vi "Map Image.vi"(2 "End of Canon highet [meters]":dbl, 3 "Goal Number":i32(knob) scale=1.0..5.0, 4 "Y[Pixels]":dbl, 5 "X [Pixels]":dbl) -> (0 "Distance [Meter]":dbl, 1 "Angel [Degrees]":dbl)   [LabVIEW 2012]
panel:
  out "Distance on ground [Meter]":dbl
  # "Goals Hights:\n1-high\n2-right\n3-left\n4-low\n5-pyramid"
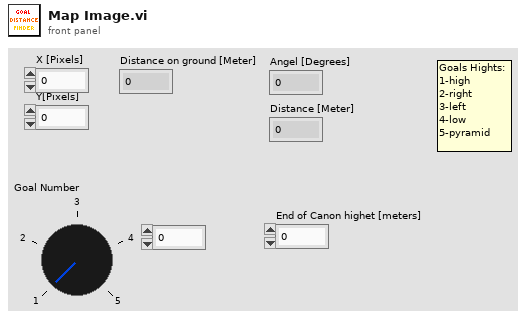
[diagram p1: front panel]
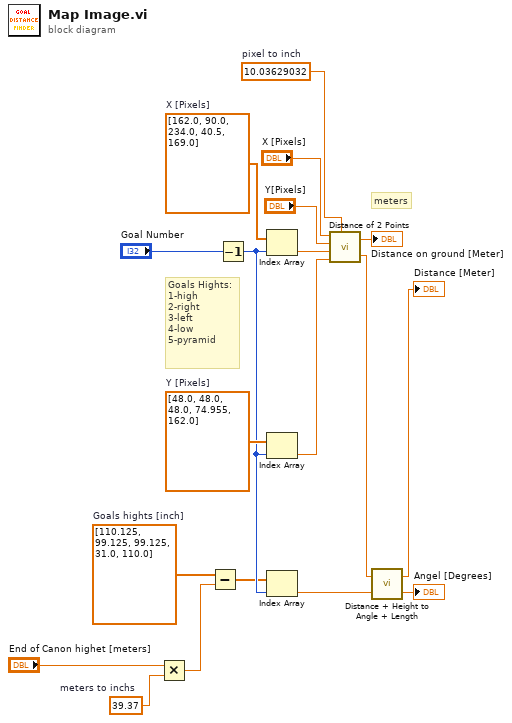
[diagram p0: block diagram]
diagram:
  w4 = 39.37  # meters to inchs
  w15 = dbl[] [48.0, 48.0, 48.0, 74.955, 162.0]  # Y [Pixels]
  w16 = dbl[] [162.0, 90.0, 234.0, 40.5, 169.0]  # X [Pixels]
  w3 = dbl[] [110.125, 99.125, 99.125, 31.0, 110.0]  # Goals hights [inch]
  w13 = 10.03629032  # pixel to inch
  # "Goals Hights:\n1-high\n2-right\n3-left\n4-low\n5-pyramid"
  # "meters"
  n1 = Multiply(x="End of Canon highet [meters]", y=w4) -> (x*y=w2:dbl)
  n2 = Subtract(x=w3, y=w2) -> (x-y=w1:dbl[])
  n3 = Decrement(x="Goal Number") -> (x-1=w6:i32)
  n4 = Index Array(array=w16, index=w6) -> (element=w7:dbl)
  n5 = Index Array(array=w15, index=w6) -> (element=w8:dbl)
  n6 = Index Array(array=w1, index=w6) -> (element=w17:dbl)
  n7 = call "Distance of 2 Points.vi"("X [Pixels]"="X [Pixels]", "Y [Pixels]"="Y[Pixels]", "X of point [Pixels]"=w7, "Y of point [Pixels]"=w8, "Conversion ratio (X*pixels = 1 * inch)"=w13) -> ("Distance on ground [Meters]"=→"Distance on ground [Meter]":dbl, "Distance on ground [Inches]"=w12:dbl)
  n8 = call "Distance + Height to Angle + Length.vi"("Highet [Inch]"=w17, "Distance on ground [Inch]"=w12) -> ("Angle [Degrees]"=→"Angel [Degrees]":dbl, "Distance[Meter]"=→"Distance [Meter]":dbl)
